vi "Generate RX Command.vi"(4 "AntennaTX4":i32, 5 "AntennaTX3":i32, 6 "AntennaTX2":i32, 7 "AntennaTX1":i32=1, 8 "RxPwrDbm":dbl=17.0, 9 "Bandwidth":string="Legacy", 10 "DataRate":string="54Mbps", 11 "Freq":i32=2412) -> (0 "rateHT40":i32, 1 "rateHT20":i32, 2 "rateLegacy":i32=128, 3 "RXCommand":string="rx f=5180; r=vt0;  pc=100; ch=0x1; macrx=01.00.00.C0.FF.EE; mactx=01.00.00.C0.FF.EE; bssid=01.00.00.C0.FF.EE; pl=1500; bc=1; ifs=1;")   [LabVIEW 2012]
panel:
  in  "VHT20 VHT40 VHT80":string[](array[string])=["MCS0", "MCS1", "MCS2", "MCS3", "MCS4", "MCS5", "MCS6", "MCS7", "MCS8", "MCS9", "MCS10", "MCS11", "MCS12", "MCS13", "MCS14", "MCS15", "MCS16", "MCS17", "MCS18", "MCS19", "MCS20", "MCS21", "MCS22", "MCS23", "MCS24", "MCS25", "MCS26", "MCS27", "MCS28", "MCS29"]
  in  "HT20HT40DataRateArray":string[](array[string])=["MCS0", "MCS1", "MCS2", "MCS3", "MCS4", "MCS5", "MCS6", "MCS7", "MCS8", "MCS9", "MCS10", "MCS11", "MCS12", "MCS13", "MCS14", "MCS15", "MCS16", "MCS17", "MCS18", "MCS19", "MCS20", "MCS21", "MCS22", "MCS23"]
  in  "LegacyDataRateArray":string[](array[string])=["6Mbps", "9Mbps", "12Mbps", "18Mbps", "24Mbps", "36Mbps", "48Mbps", "54Mbps", "1Mbps", "2Mbps-L", "2Mbps-S", "5Mbps-L", "5Mbps-S", "11Mbps-L", "11Mbps-S"]
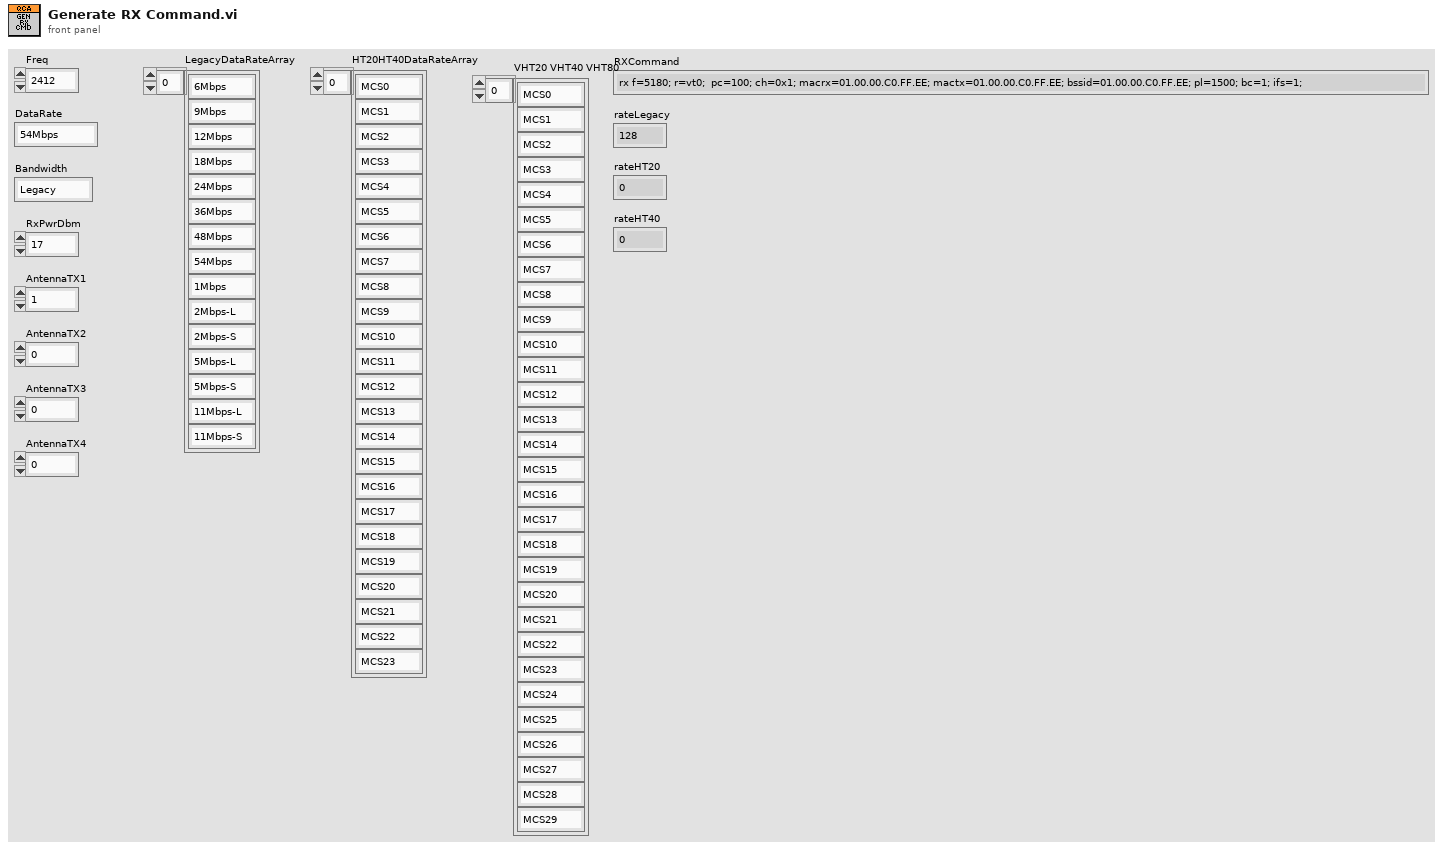
[diagram p1: front panel]
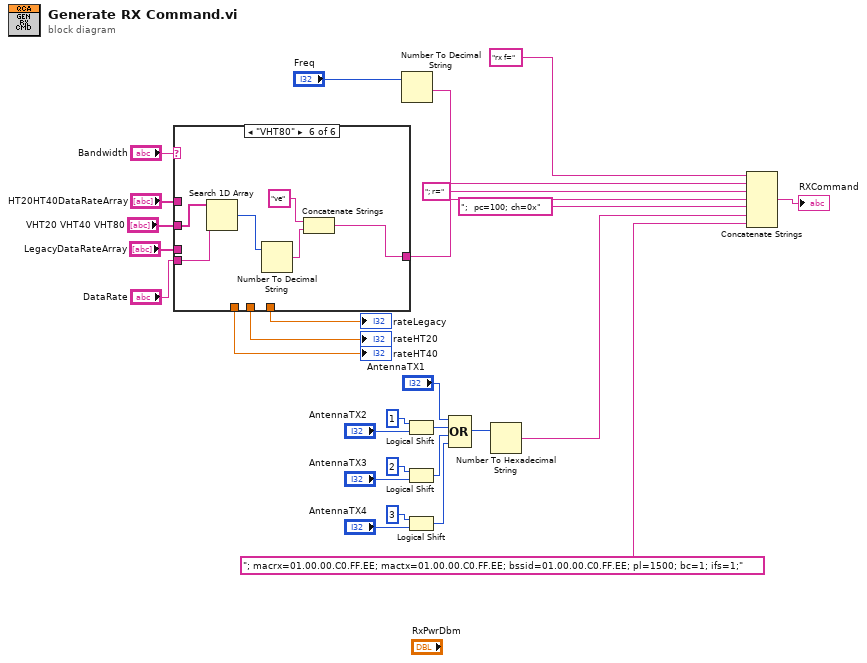
[diagram p0: block diagram]
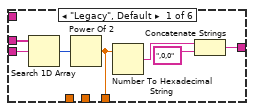
[diagram p2: hidden frame]
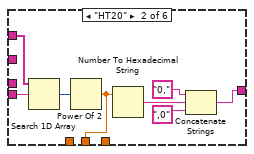
[diagram p3: hidden frame]
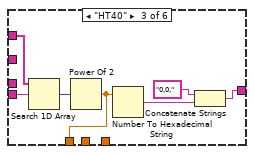
[diagram p4: hidden frame]
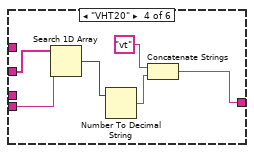
[diagram p5: hidden frame]
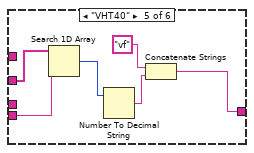
[diagram p6: hidden frame]
diagram:
  n1 = case shown="\"VHT80\"" "Bandwidth" {
    tunnel: "DataRate" -> [w34 w41 w48 w52 w58 w65]
    tunnel: "HT20HT40DataRateArray" -> [_ w42 w49 _ _ _]
    tunnel: "LegacyDataRateArray" -> [w33 _ _ _ _ _]
    tunnel: [w30 w37 w45 w53 w59 w63] -> w9
    tunnel: [w29 _ _ _ _ _] -> w5
    tunnel: [_ w36 _ _ _ _] -> w4
    tunnel: [_ _ w44 _ _ _] -> w3
    tunnel: "VHT20 VHT40 VHT80" -> [_ _ _ w51 w57 w64]
    frame "Legacy", Default {
      n2 = Search 1D Array(1D array=w33, element=w34) -> (index of element=w35:i32)  [unwired: 1 in]
      n3 = Power Of 2(x=w35) -> (2^x=w29:dbl)
      n4 = Number To Hexadecimal String(2:w29) -> (0:w32:string)  [unwired: 1 in]
      n5 = Concatenate Strings(w32, ",0,0" ("string")) -> (w30:string)
    }
    frame "HT20" {
      n6 = Search 1D Array(1D array=w42, element=w41) -> (index of element=w43:i32)  [unwired: 1 in]
      n7 = Power Of 2(x=w43) -> (2^x=w36:dbl)
      n8 = Number To Hexadecimal String(2:w36) -> (0:w40:string)  [unwired: 1 in]
      n9 = Concatenate Strings("0," ("string"), w40, ",0" ("string")) -> (w37:string)
    }
    frame "HT40" {
      n10 = Search 1D Array(1D array=w49, element=w48) -> (index of element=w50:i32)  [unwired: 1 in]
      n11 = Power Of 2(x=w50) -> (2^x=w44:dbl)
      n12 = Number To Hexadecimal String(2:w44) -> (0:w47:string)  [unwired: 1 in]
      n13 = Concatenate Strings("0,0," ("string"), w47) -> (w45:string)
    }
    frame "VHT20" {
      n14 = Search 1D Array(1D array=w51, element=w52) -> (index of element=w54:i32)  [unwired: 1 in]
      n15 = Number To Decimal String(number=w54) -> (decimal integer string=w55:string)  [unwired: 1 in]
      n16 = Concatenate Strings("vt" ("string"), w55) -> (w53:string)
    }
    frame "VHT40" {
      n17 = Search 1D Array(1D array=w57, element=w58) -> (index of element=w60:i32)  [unwired: 1 in]
      n18 = Number To Decimal String(number=w60) -> (decimal integer string=w61:string)  [unwired: 1 in]
      n19 = Concatenate Strings("vf" ("string"), w61) -> (w59:string)
    }
    frame "VHT80" {
      n20 = Search 1D Array(1D array=w64, element=w65) -> (index of element=w66:i32)  [unwired: 1 in]
      n21 = Number To Decimal String(number=w66) -> (decimal integer string=w67:string)  [unwired: 1 in]
      n22 = Concatenate Strings("ve" ("string"), w67) -> (w63:string)
    }
  }
  "rateLegacy" <- w5
  "rateHT20" <- w4
  "rateHT40" <- w3
  n23 = Number To Decimal String(number="Freq") -> (decimal integer string=w11:string)  [unwired: 1 in]
  n24 = Logical Shift(y=i8 1, x="AntennaTX2") -> (x << y=w17:i32)
  n25 = Logical Shift(y=i8 2, x="AntennaTX3") -> (x << y=w18:i32)
  n26 = Logical Shift(y=i8 3, x="AntennaTX4") -> (x << y=w19:i32)
  n27 = Compound Arithmetic op=OR("AntennaTX1", w17, w18, w19) -> (w15:i32)
  n28 = Number To Hexadecimal String(2:w15) -> (0:w7:string)  [unwired: 1 in]
  n29 = Concatenate Strings("rx f=" ("string"), w11, "; r=" ("string"), w9, ";  pc=100; ch=0x" ("string"), w7, "; macrx=01.00.00.C0.FF.EE; mactx=01.00.00.C0.FF.EE; bssid=01.00.00.C0.FF.EE; pl=1500; bc=1; ifs=1;" ("string")) -> (→"RXCommand":string)
